vi "Global .vi"() -> ()   [LabVIEW 2022 SP3]
panel:
  out "Stop":bool
  in  "ECU TYPE":u16(ring)
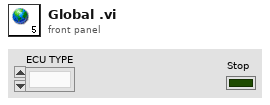
[diagram p1: front panel]
diagram:
